vi "Case_Structure2.vi"() -> ()   [LabVIEW 2022 SP3]
panel:
  out "String 3":string
  in  "String 2":string
  out "String":string
  in  "Numeric":i32
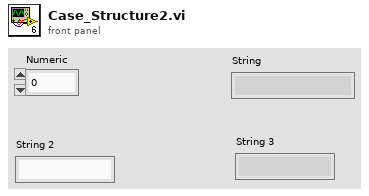
[diagram p1: front panel]
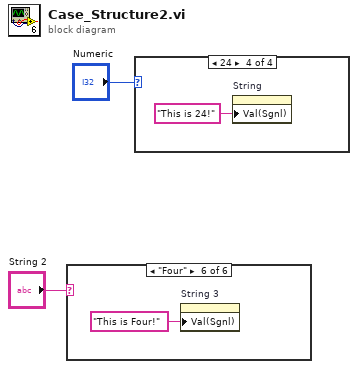
[diagram p0: block diagram]
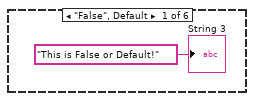
[diagram p2: hidden frame]
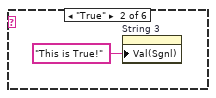
[diagram p3: hidden frame]
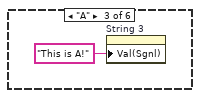
[diagram p4: hidden frame]
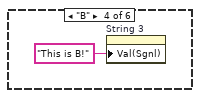
[diagram p5: hidden frame]
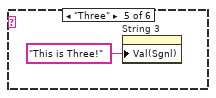
[diagram p6: hidden frame]
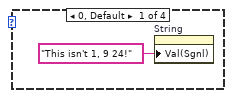
[diagram p7: hidden frame]
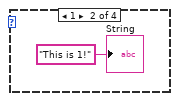
[diagram p8: hidden frame]
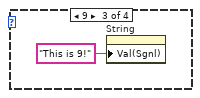
[diagram p9: hidden frame]
diagram:
  n1 = case shown="\"Four\"" "String 2" {
    frame "False", Default {
      "String 3" <- "This is False or Default!" ("String 3")
    }
    frame "True" {
      n2 = property on="String 3" class="Str"("Val(Sgnl)"="This is True!" ("Value (Signaling)")) -> ()  [unwired: 2 in, 2 out]
    }
    frame "A" {
      n3 = property on="String 3" class="Str"("Val(Sgnl)"="This is A!" ("Value (Signaling)")) -> ()  [unwired: 2 in, 2 out]
    }
    frame "B" {
      n4 = property on="String 3" class="Str"("Val(Sgnl)"="This is B!" ("Value (Signaling)")) -> ()  [unwired: 2 in, 2 out]
    }
    frame "Three" {
      n5 = property on="String 3" class="Str"("Val(Sgnl)"="This is Three!" ("Value (Signaling)")) -> ()  [unwired: 2 in, 2 out]
    }
    frame "Four" {
      n6 = property on="String 3" class="Str"("Val(Sgnl)"="This is Four!" ("Value (Signaling)")) -> ()  [unwired: 2 in, 2 out]
    }
  }
  n7 = case shown="24" "Numeric" {
    frame 0, Default {
      n8 = property on="String" class="Str"("Val(Sgnl)"="This isn't 1, 9 24!" ("Value (Signaling)")) -> ()  [unwired: 2 in, 2 out]
    }
    frame 1 {
      "String" <- "This is 1!" ("String")
    }
    frame 9 {
      n9 = property on="String" class="Str"("Val(Sgnl)"="This is 9!" ("Value (Signaling)")) -> ()  [unwired: 2 in, 2 out]
    }
    frame 24 {
      n10 = property on="String" class="Str"("Val(Sgnl)"="This is 24!" ("Value (Signaling)")) -> ()  [unwired: 2 in, 2 out]
    }
  }
